vi "Log Data.vi"(8 "error in (no error)":errorcluster, 9 "Logging?":bool, 10 "Channels to log":bool[](array[boolean]), 11 "Array":dbl[][](array[numeric])) -> (0 "error out":errorcluster)   [LabVIEW 2020]
doc: "writes the selected channels to disk."
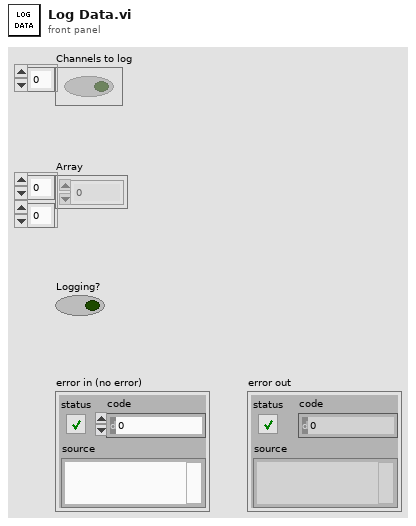
[diagram p1: front panel]
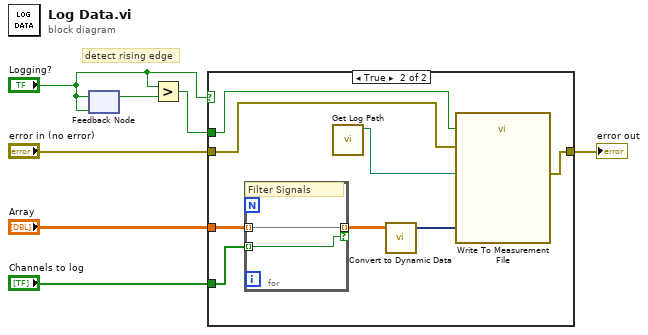
[diagram p0: block diagram]
diagram:
  # "detect rising edge"
  n1 = feedback #1("Logging?") -> (w3:bool)
  n2 = feedback-in #1("Logging?") -> ()
  n3 = Greater?(x="Logging?", y=w3) -> (0:w1:bool)
  n4 = case shown="True" "Logging?" {
    tunnel: [w8 w15] -> w7
    tunnel: "error in (no error)" -> [w8 w14]
    tunnel: "Array" -> [_ w13]
    tunnel: "Channels to log" -> [_ w11]
    tunnel: w1 -> [_ w10]
    frame False {
    }
    frame True {
      n5 = for {
        tunnel: w13 -> [w18] mode=indexing
        tunnel: [w18] -> w12 mode=indexing if=w17
        tunnel: w11 -> [w17] mode=indexing
        # "Filter Signals"
      }
      n6 = call "Get Log Path.vi"() -> ("appended path"=w9:path)  [unwired: 11 in]
      n7 = call "Convert to Dynamic Data"("2D Array"=w12) -> ("Dynamic Data Type"=w16:dynamicdata)  [unwired: 3 in]
      n8 = call "Write To Measurement File"("Signals"=w16, "Reset"=w10, "error in (no error)"=w14, "Filename"=w9) -> ("error out"=w15:errorcluster)  [unwired: 13 in, 2 out]
    }
  }
  "error out" <- w7
